vi "ReloadCSVforanalysispart_171213.vi"(0 "Path":path) -> (1 "Whole dataset array":dbl[][](array[numeric]), 3 "Clean data array":dbl[][](array[numeric]), 4 "Errors array":dbl[][](array[numeric]), 5 "Number of errors":i32, 6 "Time":string[](array[string]))   [LabVIEW 2016]
uses:
  <vilib>/Utility/file.llb/Read Delimited Spreadsheet (DBL).vi
  <vilib>/Utility/file.llb/Read Delimited Spreadsheet (string).vi
panel:
  out "all rows":string[][](array[string])
  out "first row":string[](array[string])
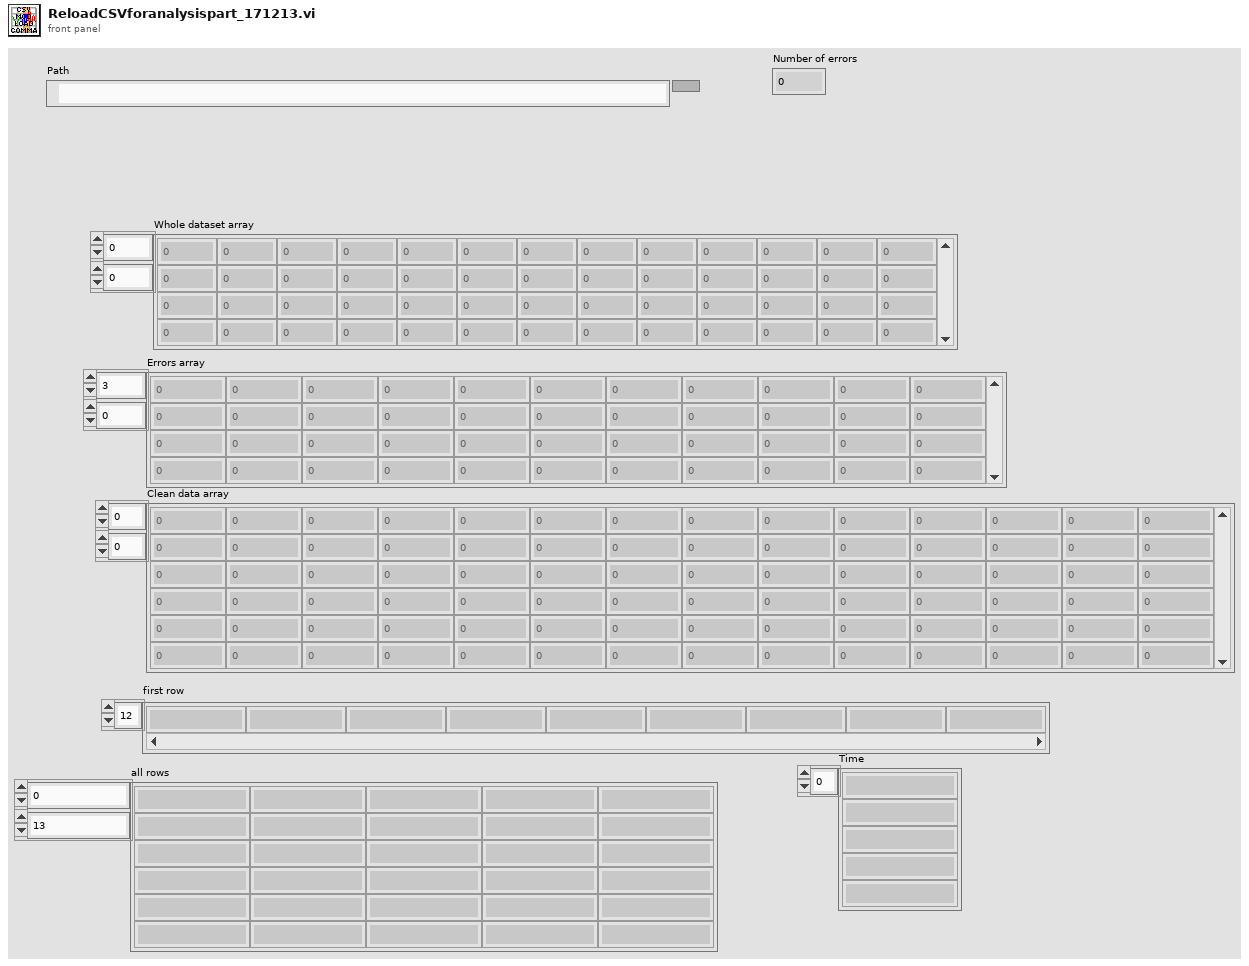
[diagram p1: front panel]
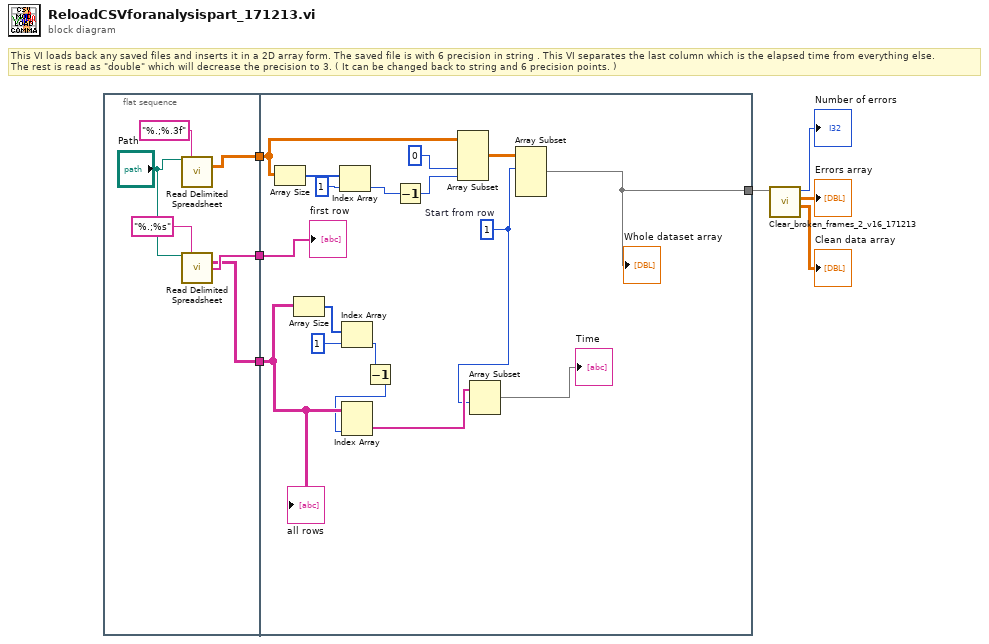
[diagram p0: block diagram]
diagram:
  # "This VI loads back any saved files and inserts it in a 2D array form. The saved file is with 6 precision in string . This VI separates the last column which is the elapsed time from everything else.\nThe rest is read as \"double\" which will decrease the precision to 3. ( It can be changed back to string and 6 precision points. )"
  n1 = flat-sequence {
    tunnel: [w13] -> w7
    tunnel: [w11] -> w6
    tunnel: [w10] -> w5
    tunnel: [w26] -> w4
    tunnel: w7 -> [w18]
    tunnel: w6 -> [w24]
    tunnel: w5 -> [w20]
    frame #0 {
      n2 = call-poly <vilib>:"Read Delimited Spreadsheet.vi"("file path (dialog if empty)"="Path", "format (%.3f)"="%.;%.3f") -> ("all rows"=w13:dbl[][])  [unwired: 8 in, 5 out]
      n3 = call-poly <vilib>:"Read Delimited Spreadsheet.vi"("file path (dialog if empty)"="Path", "format (%s)"="%.;%s") -> ("all rows"=w10:string[][], "first row"=w11:string[])  [unwired: 8 in, 4 out]
    }
    frame #1 {
      w16 = 1  # Start from row
      n4 = Array Size(array=w18) -> (size(s)=w30:i32[])
      n5 = Array Size(array=w20) -> (size(s)=w23:i32[])
      n6 = Index Array(array=w30, index=1) -> (element=w25:i32)
      n7 = Index Array(array=w23, index=1) -> (element=w21:i32)
      n8 = Decrement(x=w21) -> (x-1=w14:i32)
      n9 = Index Array(array=w20, index (col)=w14) -> (element=w17:string[])  [unwired: 1 in]
      n10 = Decrement(x=w25) -> (x-1=w19:i32)
      n11 = Array Subset(array=w18, index (col)=0 ("index"), length (col)=w19) -> (w27:dbl[][])  [unwired: 2 in]
      n12 = Array Subset(array=w17, index=w16) -> (→"Time":string[])  [unwired: 1 in]
      n13 = Array Subset(array=w27, index (row)=w16) -> (w26:dbl[][])  [unwired: 3 in]
      "Whole dataset array" <- w26
      "first row" <- w24
      "all rows" <- w20
    }
  }
  n14 = call "Clear_broken_frames_2_v16_171213.vi"("Input  data 2D array"=w4) -> ("Cleaned array"=→"Clean data array":dbl[][], "Errors array"=→"Errors array":dbl[][], "Number of errors"=→"Number of errors":i32)  [unwired: 8 in]
